vi "Getdb_ref_array.vi"(8 "error in (no error)":errorcluster, 11 "OneOfTemplate in":refnum<class "nixnet_grpc_DbGetPropertyResponse_property_value.lvclass">) -> (0 "error out":errorcluster, 2 "Get_Val":T1, 3 "OneOfTemplate out":refnum<class "nixnet_grpc_DbGetPropertyResponse_property_value.lvclass">)   [LabVIEW 2019, in "xnet-grpc_client.lvlib" / "nixnet_grpc_DbGetPropertyResponse_property_value.lvclass"]
uses:
  nixnet_grpc_DbGetPropertyResponse_property_value.lvclass
  nixnet_grpc_DbRefArray.ctl
  nidevice_grpc_Session.ctl
  nixnet_grpc_DbGetPropertyResponse_property_value.lvclass/nixnet_grpc_DbGetPropertyResponse_property_value.ctl
  xnet-grpc_client.lvlib
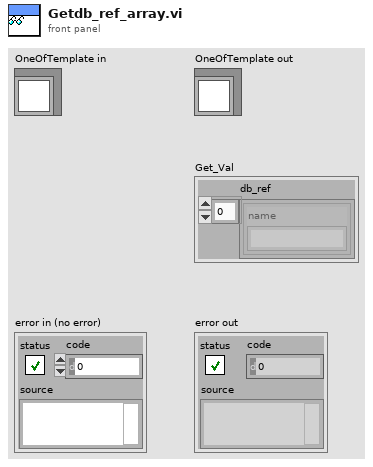
[diagram p1: front panel]
types:
  T1 = typedef "xnet-grpc_client.lvlib/nixnet_grpc_DbRefArray.ctl" = cluster{"db_ref":T2[]}
  T2 = typedef "xnet-grpc_client.lvlib/nidevice_grpc_Session.ctl" = cluster{"name":string}
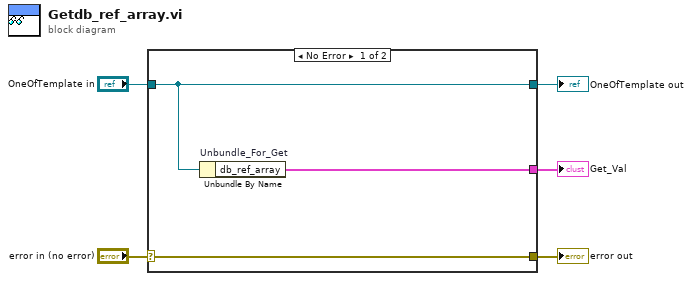
[diagram p0: block diagram]
diagram:
  n1 = case shown="No Error" "error in (no error)" {
    selector: "error in (no error)" -> [w8 w9]
    tunnel: [w8 w9] -> w4
    tunnel: [w7 w10] -> w2
    tunnel: "OneOfTemplate in" -> [w7 w10]
    tunnel: [w6 _] -> w1
    frame No Error {
      n2 = Unbundle By Name "Unbundle_For_Get"(w7) -> ("db_ref_array"=w6:T1)
    }
    frame Error {
    }
  }
  "error out" <- w4
  "OneOfTemplate out" <- w2
  "Get_Val" <- w1
